vi "Color Histogram.vi"() -> ()   [LabVIEW 2014]
doc: "Use this template to build a VI to use as a subVI."
uses:
  <vilib>/vision/NI_Vision_Development_Module.lvlib
panel:
  out "Histogram-V":T1(graph)
  out "Histogram-S":T1(graph)
  out "Histogram-H":T1(graph)
  out "Src":T2(plugin-control)
  # ":: MVi Framework V1.0 ::\nAuthor:Gaoke Yang\nEmail: gaoke.yang@yahoo.com\nWeb: www.mvicontrol.com\nCopyright (C) 2015, MVI Technologies All Rights Reserved"
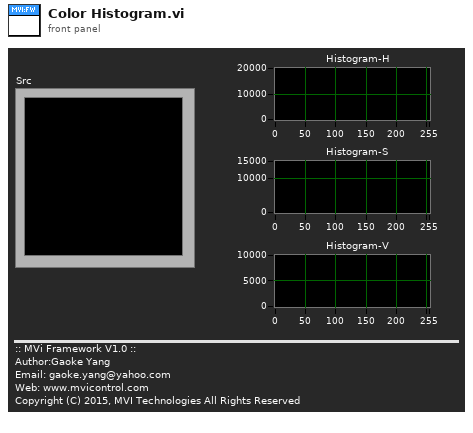
[diagram p1: front panel]
types:
  T1 = cluster{"Starting Value":sgl, "Incremental Value":sgl, "Histogram":u32[]}
  T2 = typedef "IMAQ Image.ctl" = refnum<image>
  T3 = typedef "Image Type" = u32
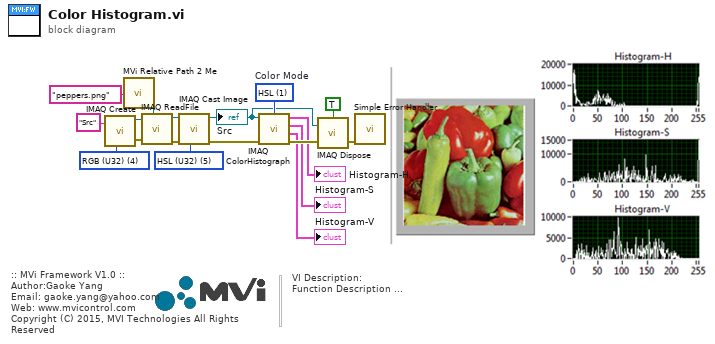
[diagram p0: block diagram]
diagram:
  w4 = T3 4 items=["Grayscale (U8)", "Grayscale (I16)", "Grayscale (SGL)", "Complex (CSG)", "RGB (U32)", "HSL (U32)", "RGB (U64)", "Grayscale (U16)"] ("Image Type")
  w7 = u16 1 items=["RGB", "HSL", "HSV", "HSI"]  # Color Mode
  w9 = T3 5 items=["Grayscale (U8)", "Grayscale (I16)", "Grayscale (SGL)", "Complex (CSG)", "RGB (U32)", "HSL (U32)", "RGB (U64)", "Grayscale (U16)"] ("Image Type")
  # "VI Description:\nFunction Description ..."
  # ":: MVi Framework V1.0 ::\nAuthor:Gaoke Yang\nEmail: gaoke.yang@yahoo.com\nWeb: www.mvicontrol.com\nCopyright (C) 2015, MVI Technologies All Rights Reserved"
  n1 = call "IMAQ Create"("Image Name"="Src" ("name or relative path"), "Image Type"=w4) -> ("New Image"=w13:T2, "error out"=w12:errorcluster)  [unwired: 2 in, 1 out]
  n2 = call "MVi Relative Path 2 Me.vi"("Relative Path"="peppers.png" ("name or relative path")) -> ("Appended Dir"=w14:path)  [unwired: 5 in, 1 out]
  n3 = call "IMAQ ReadFile"("File Path"=w14, "error in (no error)"=w12, "Image"=w13) -> ("error out"=w11:errorcluster, "Image Out"=w10:T2)  [unwired: 4 in, 3 out]
  n4 = call "IMAQ Cast Image"("Image Type"=w9, "error in (no error)"=w11, "Image Src"=w10) -> ("error out"=w8:errorcluster, "Image Dst Out"=w5:T2)  [unwired: 7 in]
  "Src" <- w5
  n5 = call "IMAQ ColorHistograph"("Color Mode"=w7, "Image Src"=w5, "error in (no error)"=w8) -> ("Red or Hue Histogram Graph"=→"Histogram-H":T1, "Green or Sat Histogram Graph"=→"Histogram-S":T1, "Blue or Luma or Val or Inten Histogram Graph"=→"Histogram-V":T1, "error out"=w6:errorcluster)  [unwired: 3 in]
  n6 = call "IMAQ Dispose"("All Images? (No)"=TRUE, "Image"=w5, "error in (no error)"=w6) -> ("error out"=w15:errorcluster)  [unwired: 3 out]
  n7 = call <vilib>:"Simple Error Handler.vi"("error in (no error)"=w15) -> ()  [unwired: 1 in, 8 out]
